vi "DeadZone.vi"(1 "Drive Axes":cluster{"X axis":dbl, "Y axis":dbl}) -> (0 "Drive Axes":cluster{"X axis":dbl, "Y axis":dbl})   [LabVIEW 2014]
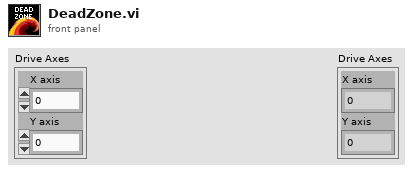
[diagram p1: front panel]
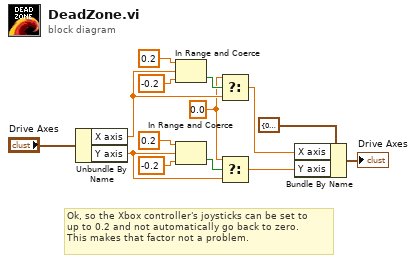
[diagram p0: block diagram]
diagram:
  w7 = 0.0 ("t")
  # "Ok, so the Xbox controller's joysticks can be set to \nup to 0.2 and not automatically go back to zero.\nThis makes that factor not a problem."
  n1 = Unbundle By Name("Drive Axes") -> ("X axis"=w8:dbl, "Y axis"=w6:dbl)
  n2 = In Range and Coerce(upper limit=0.2, x=w8, lower limit=-0.2) -> (In Range?=w9:bool)  [unwired: 1 out]
  n3 = In Range and Coerce(upper limit=0.2, x=w6, lower limit=-0.2) -> (In Range?=w5:bool)  [unwired: 1 out]
  n4 = Select(t=w7, s=w9, f=w8) -> (s? t:f=w3:dbl)
  n5 = Select(t=w7, s=w5, f=w6) -> (s? t:f=w2:dbl)
  n6 = Bundle By Name(cluster=cluster{"X axis":dbl, "Y axis":dbl} {"X axis"=0.0, "Y axis"=0.0} ("Drive Axes 2"), "X axis"=w3, "Y axis"=w2) -> (→"Drive Axes":cluster{"X axis":dbl, "Y axis":dbl})
